vi "get information display strings.vi"(8 "error in":errorcluster, 11 "NISE_CEF_serializable node in":refnum<class "NISE_CEF_serializable node.lvclass">) -> (0 "error out":errorcluster, 1 "Data":string[](array[string]), 2 "Labels":string[](array[string]), 3 "NISE_CEF_serializable node out":refnum<class "NISE_CEF_serializable node.lvclass">)   [LabVIEW 2013, in "NISE_CEF_serializable node.lvclass"]
uses:
  NISE_CEF_serializable node.lvclass
  serializable configuration/NISE_CEF_serializable configuration.lvclass/NISE_CEF_serializable configuration.ctl
  serializable configuration/NISE_CEF_serializable configuration.lvclass
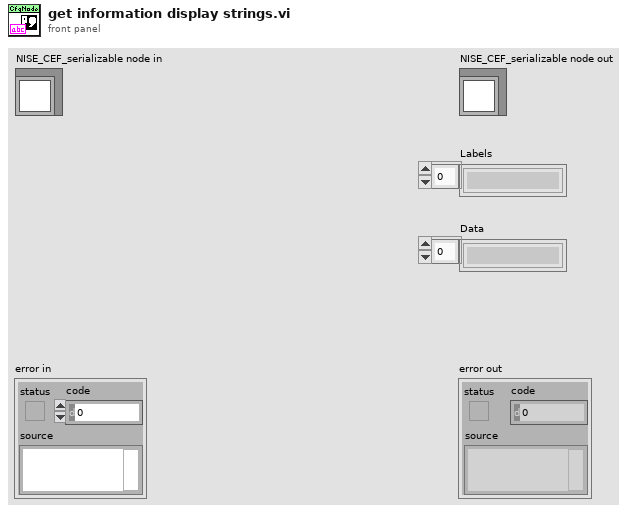
[diagram p1: front panel]
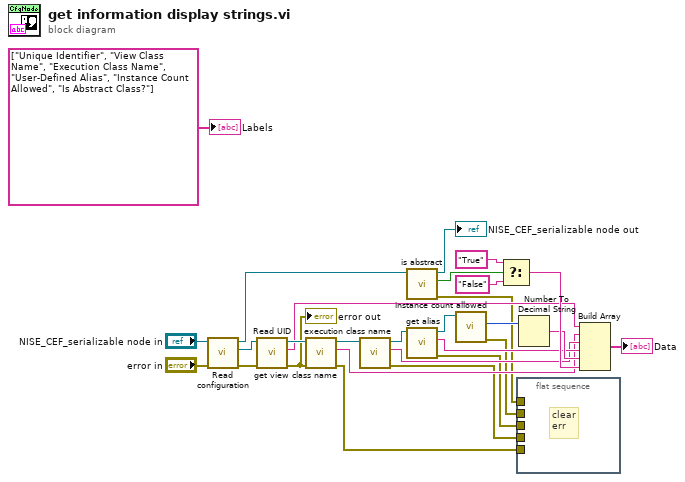
[diagram p0: block diagram]
diagram:
  n1 = call-dynamic "Read configuration.vi"("error in"="error in", "NISE_CEF_serializable node in"="NISE_CEF_serializable node in") -> ("error out"=w19:errorcluster, "configuration"=w20:refnum<class "NISE_CEF_serializable configuration.lvclass">, "NISE_CEF_serializable node out"=w25:refnum<class "NISE_CEF_serializable node.lvclass">)  [unwired: 7 in]
  n2 = call "Read UID.vi"("error in"=w19, "configuration in"=w20) -> ("error out"=w6:errorcluster, "instance id"=w7:string, "configuration out"=w24:refnum<class "NISE_CEF_serializable configuration.lvclass">)  [unwired: 7 in]
  "error out" <- w6
  n3 = call "get view class name.vi"("error in"=w6, "configuration in"=w24) -> ("error out"=w5:errorcluster, "view class"=w8:string, "configuration out"=w23:refnum<class "NISE_CEF_serializable configuration.lvclass">)  [unwired: 7 in]
  n4 = call-dynamic "execution class name.vi"("configuration in"=w23) -> ("error out"=w4:errorcluster, "execution class"=w9:string, "configuration out"=w22:refnum<class "NISE_CEF_serializable configuration.lvclass">)  [unwired: 8 in]
  n5 = call-dynamic "is abstract.vi"("NISE_CEF_serializable node in"=w25) -> ("error out"=w1:errorcluster, "abstract"=w17:bool, "NISE_CEF_serializable node out"=→"NISE_CEF_serializable node out":refnum<class "NISE_CEF_serializable node.lvclass">)  [unwired: 8 in]
  n6 = call "get alias.vi"("configuration in"=w22) -> ("error out"=w3:errorcluster, "alias"=w10:string, "configuration out"=w21:refnum<class "NISE_CEF_serializable configuration.lvclass">)  [unwired: 8 in]
  n7 = call-dynamic "instance count allowed.vi"("configuration in"=w21) -> ("error out"=w2:errorcluster, "instances allowed"=w12:i32)  [unwired: 8 in, 1 out]
  n8 = Select(t="True", s=w17, f="False") -> (s? t:f=w14:string)
  n9 = flat-sequence {
    tunnel: w5 -> [_]
    tunnel: w4 -> [_]
    tunnel: w3 -> [_]
    tunnel: w2 -> [_]
    tunnel: w1 -> [_]
    frame #0 {
      # "clear\nerr"
    }
  }
  n10 = Number To Decimal String(number=w12) -> (decimal integer string=w11:string)  [unwired: 1 in]
  n11 = Build Array(w7, w8, w9, w10, w11, w14) -> (→"Data":string[])
  "Labels" <- string[] ["Unique Identifier", "View Class Name", "Execution Class Name", "User-Defined Alias", "Instance Count Allowed", "Is Abstract Class?"] ("Labels")
